vi "Initialize.vi"(7 "ChannelName":string="Setpoint.ch%d.SP", 8 "error in":errorcluster, 9 "Number of Channels":u32=1, 10 "Instance Name":string="PluginName", 11 "Power Gradient in":refnum<class "Power Gradient.lvclass">) -> (0 "error out":errorcluster, 3 "Power Gradient out":refnum<class "Power Gradient.lvclass">)   [LabVIEW 2023, in "Power Gradient.lvclass"]
uses:
  Power Gradient.lvclass
  Power Gradient.lvclass/Power Gradient.ctl
  Parents/Gradient/Gradient.lvclass
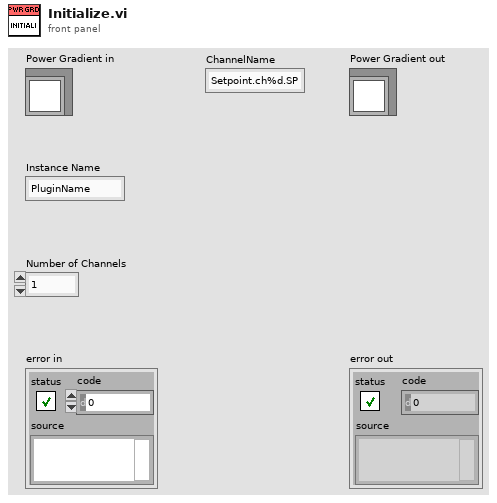
[diagram p1: front panel]
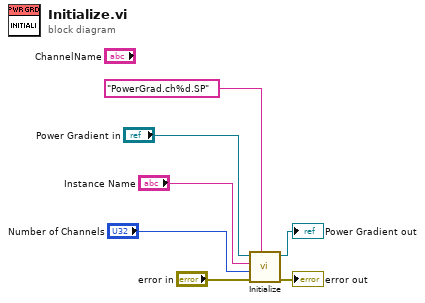
[diagram p0: block diagram]
diagram:
  n1 = call-parent "Initialize.vi"("ChannelName"="PowerGrad.ch%d.SP", "error in"="error in", "Number of Channels"="Number of Channels", "Instance Name"="Instance Name", "Gradient in"="Power Gradient in") -> ("error out"=→"error out":errorcluster, "Gradient out"=→"Power Gradient out":refnum<class "Power Gradient.lvclass">)  [unwired: 5 in]
